vi "ReadThingSpeak.vi"() -> ()   [LabVIEW 2019]
uses:
  <vilib>/httpClient/LabVIEWHTTPClient.lvlib
panel:
  out "body":string
  out "headers":string
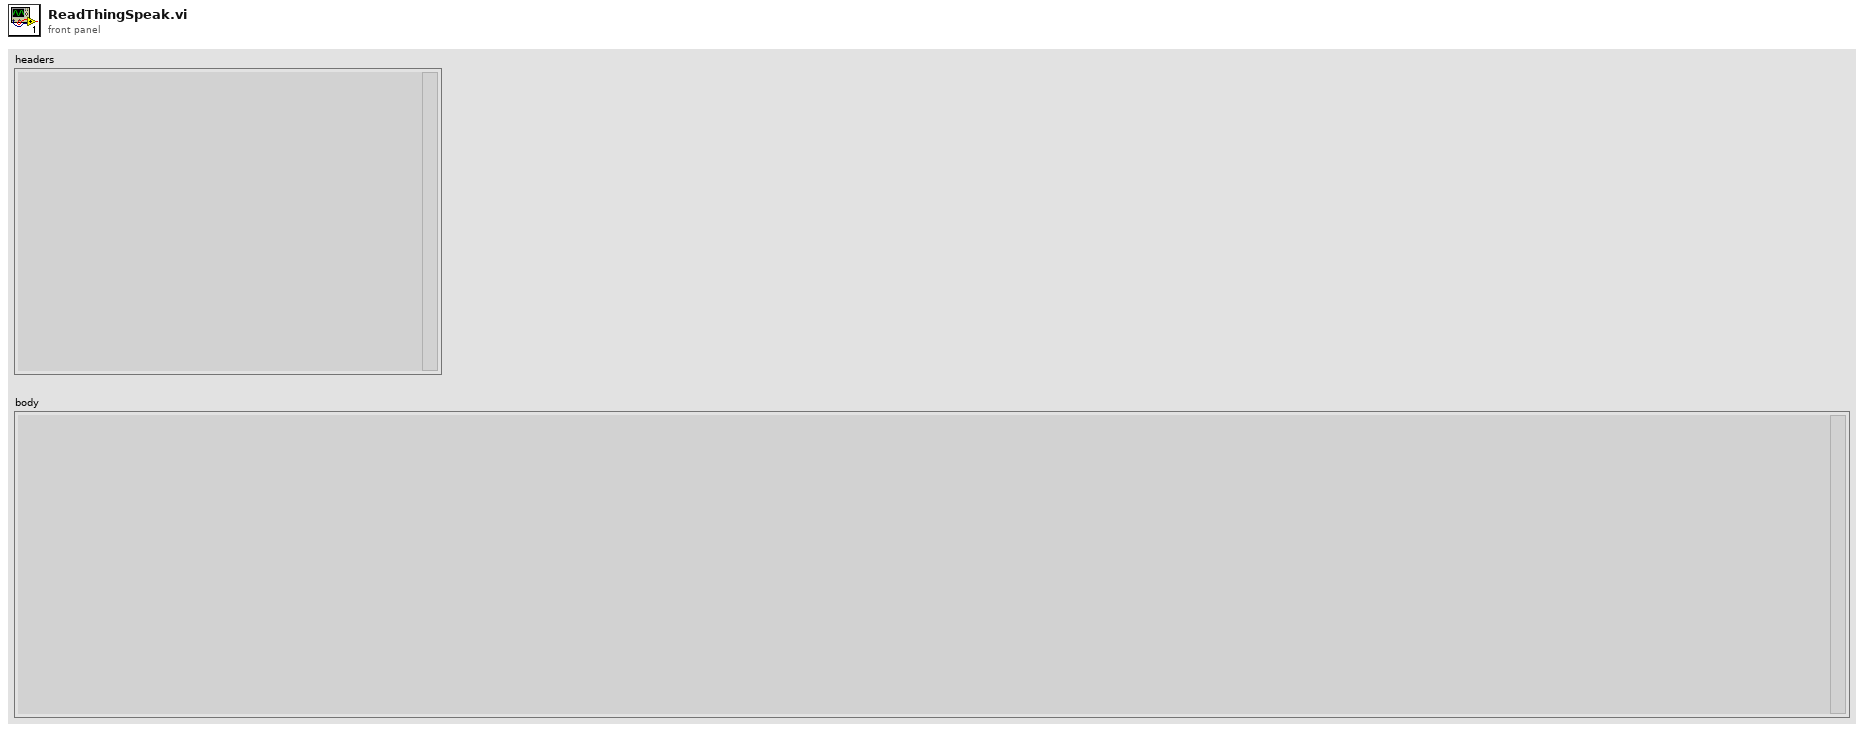
[diagram p1: front panel]
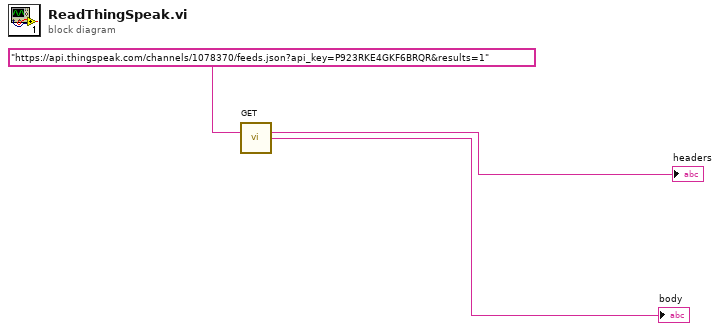
[diagram p0: block diagram]
diagram:
  n1 = call <vilib>:"GET.vi"("url"="https://api.thingspeak.com/channels/1078370/feeds.json?api_key=P923RKE4GKF6BRQR&results=1" ("format string")) -> ("headers"=→"headers":string, "body"=→"body":string)  [unwired: 11 in, 2 out]
